vi "启动采集.vi"(8 "错误输入":errorcluster caption="错误输入（无错误）", 9 "时钟源":i32, 10 "伪同步":i32, 11 "设备句柄入":i32) -> (0 "错误输出":errorcluster, 3 "设备句柄":i32=1)   [LabVIEW 2011]
uses:
  dll/em9636.dll
panel:
  in  "超时毫秒":i32=1000
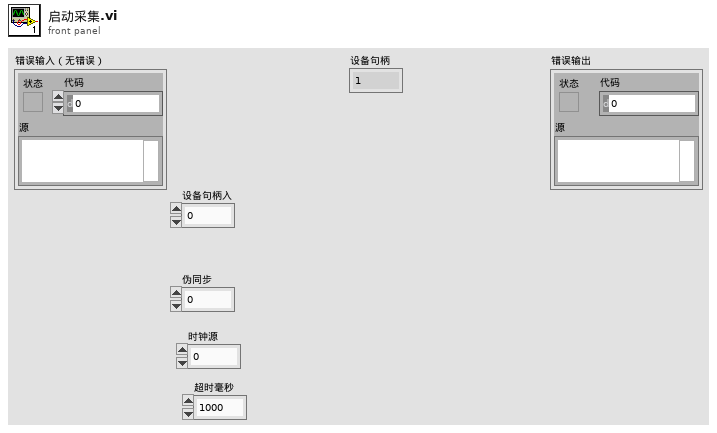
[diagram p1: front panel]
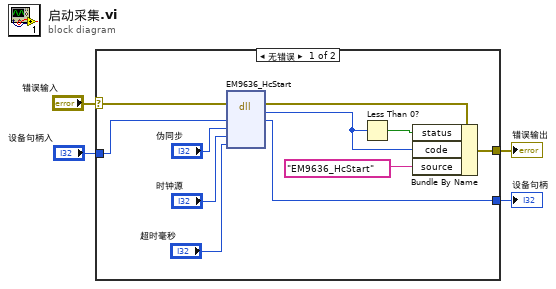
[diagram p0: block diagram]
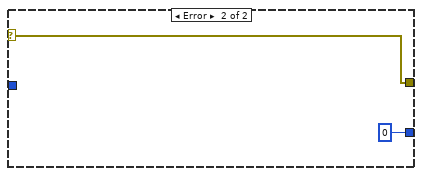
[diagram p2: hidden frame]
diagram:
  n1 = case shown="无错误" "错误输入" {
    selector: "错误输入" -> [w15 w17]
    tunnel: [w11 w17] -> w3
    tunnel: [w5 0 ("错误")] -> w2
    tunnel: "设备句柄入" -> [w9 _]
    frame No Error {
      n2 = dll-call lib="PTH1abs Eèµ éç LABVIEWæºVI(v2.0)EM9636BD)EM9636BDè°ç¨APIå½æ°æ¹æ³éè®¯ä¾ç¨EM9636labview8.5-1511048.5dll\nem9636.dll" fn="EM9636_HcStart"(error in=w15, "设备句柄"=w9, "伪同步"="伪同步", "时钟源"="时钟源", "超时毫秒"="超时毫秒") -> (error out=w13:errorcluster, "错误"=w10:i32, "设备句柄"=w5:i32)  [unwired: 5 in, 1 out]
      n3 = Less Than 0?(x=w10) -> (x < 0?=w12:bool)
      n4 = Bundle By Name(cluster=w13, "status"=w12, "code"=w10, "source"="EM9636_HcStart") -> (w11:errorcluster)
    }
    frame Error {
    }
  }
  "错误输出" <- w3
  "设备句柄" <- w2
